vi "GetCallerVIRef.vi"(10 "error in (no error)":errorcluster) -> (2 "error out":errorcluster, 3 "VI out":refnum<vi>)   [LabVIEW 2019]
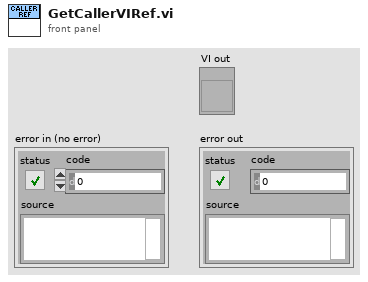
[diagram p1: front panel]
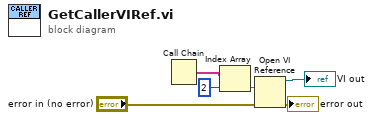
[diagram p0: block diagram]
diagram:
  n1 = Call Chain() -> (call chain=w3:string[])
  n2 = Index Array(array=w3, index=2) -> (element=w2:string)
  n3 = Open VI Reference(vi path=w2, error in (no error)="error in (no error)") -> (vi reference=→"VI out":refnum<vi>, error out=→"error out":errorcluster)  [unwired: 4 in]
